vi "Configure Test Time.vi"(7 "Mode":T2 items=["AC", "DC", "IR"], 8 "error in (no error)":errorcluster, 9 "Test Time [s]":dbl=3.0 min=0.0 max=999.0 step=0.1 format="%.1f", 10 "Step":T1=1 min=1 max=99 step=1, 11 "VISA resource name":refnum<visa-resource-name>) -> (0 "error out":errorcluster, 3 "VISA resource name out":refnum<visa-resource-name>)   [LabVIEW 2025]
uses:
  <instrlib>/Chrome 19025/Public/Utility/Type Def/AC-DC-IR modes--ring.ctl
  <instrlib>/Chrome 19025/Public/Utility/Type Def/steps--numeric.ctl
panel:
  # "Configure Test Time"
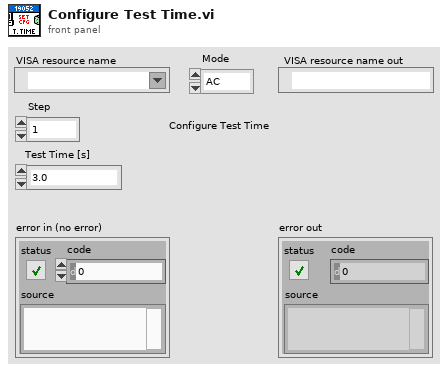
[diagram p1: front panel]
types:
  T1 = typedef "Chrome 19025.lvlib/steps--numeric.ctl" = u8
  T2 = typedef "Chrome 19025.lvlib/AC-DC-IR modes--ring.ctl" = u16
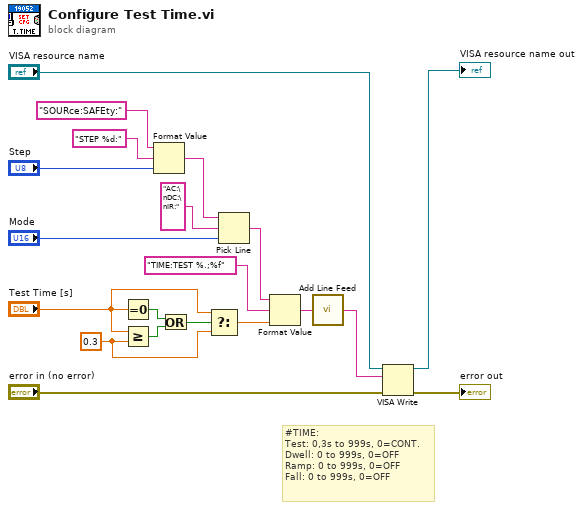
[diagram p0: block diagram]
diagram:
  w3 = 0.3 ("y")
  # "#TIME: \nTest: 0,3s to 999s, 0=CONT. \nDwell: 0 to 999s, 0=OFF\nRamp: 0 to 999s, 0=OFF\nFall: 0 to 999s, 0=OFF"
  n1 = Equal To 0?(x="Test Time [s]") -> (x = 0?=w6:bool)
  n2 = Greater Or Equal?(x="Test Time [s]", y=w3) -> (x >= y?=w5:bool)
  n3 = Format Value(string ("")="SOURce:SAFEty:", format string="STEP %d:", value (0)="Step") -> (output string=w15:string)
  n4 = Or(x=w6, y=w5) -> (x .or. y?=w4:bool)
  n5 = Select(t="Test Time [s]", s=w4, f=w3) -> (s? t:f=w1:dbl)
  n6 = Pick Line(string ("")=w15, multi-line string="AC:\nDC:\nIR:", line index="Mode") -> (output string=w13:string)
  n7 = Format Value(string ("")=w13, format string="TIME:TEST %.;%f", value (0)=w1) -> (output string=w12:string)
  n8 = call <instrlib>:"Add Line Feed.vi"("Command string"=w12) -> ("Concatenated string"=w11:string)  [unwired: 4 in]
  n9 = VISA Write(VISA resource name="VISA resource name", write buffer=w11, error in (no error)="error in (no error)") -> (VISA resource name out=→"VISA resource name out":refnum<visa-resource-name>, error out=→"error out":errorcluster)  [unwired: 1 out]
